vi "calculate timestamp microseconds.vi"(1 "timestamp in":u64 format="%x") -> (0 "timestamp out":u64)   [LabVIEW 2024, in "atsj peakcan basic.lvlib"]
uses:
  atsj peakcan basic.lvlib
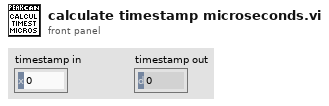
[diagram p1: front panel]
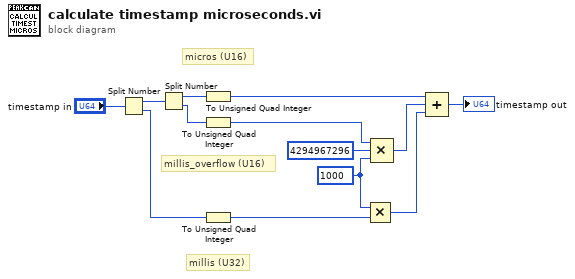
[diagram p0: block diagram]
diagram:
  w1 = u64 1000
  # "micros (U16)"
  # "millis_overflow (U16)"
  # "millis (U32)"
  n1 = Split Number(x="timestamp in") -> (hi(x)=w12:u32, lo(x)=w13:u32)
  n2 = Split Number(x=w12) -> (hi(x)=w7:u16, lo(x)=w9:u16)
  n3 = To Unsigned Quad Integer(1:w7) -> (0:w5:u64)
  n4 = To Unsigned Quad Integer(1:w9) -> (0:w8:u64)
  n5 = To Unsigned Quad Integer(1:w13) -> (0:w10:u64)
  n6 = Multiply(x=w1, y=w10) -> (x*y=w2:u64)
  n7 = Compound Arithmetic op=MULTIPLY(w8, u64 4294967296, w1) -> (w6:u64)
  n8 = Compound Arithmetic op=ADD(w5, w6, w2) -> (→"timestamp out":u64)
